vi "manual_random.vi"(8 "error in (no error)":errorcluster, 11 "data":variant) -> (0 "error out":errorcluster)   [LabVIEW 2015, in "example_01.lvlib"]
doc: "manual_random.vi will generate a random value and provide it via variant."
uses:
  example_01.lvlib
  _controls/steps_actions_data.ctl
  _controls/steps_actions.ctl
  <userlib>/antonio-alexander/lv-recipe-machine/lv-recipe-machine.lvlib
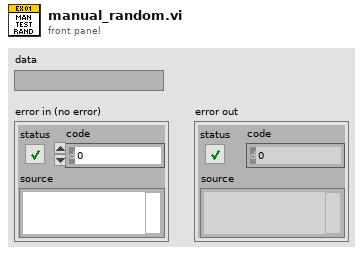
[diagram p1: front panel]
types:
  T1 = typedef "example_01.lvlib/steps_actions.ctl" = enum16{"<steps_actions>", "manual_random", "manual_comparison", "manual_wait", "auto_random", "auto_wait", "criteria_initialize", "criteria_count", "criteria_comparison", "transition_simple", "transition_count", "transition_comparison", "launch_wait", "<null>"}
  T2 = typedef "example_01.lvlib/steps_actions_data.ctl" = cluster{"step_action":T1, "data":variant}
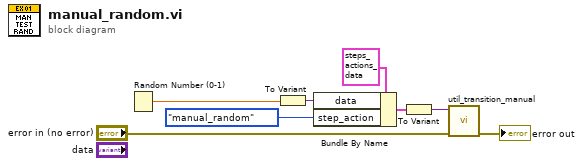
[diagram p0: block diagram]
diagram:
  n1 = Random Number (0-1)() -> (number: 0 to 1=w5:dbl)
  n2 = To Variant(anything=w5) -> (Variant=w4:variant)
  n3 = Bundle By Name(cluster=T2 {"step_action"=enum."<steps_actions>", "data"=variant}, "data"=w4, "step_action"=steps_actions."manual_random" ("manual_action")) -> (w6:T2)
  n4 = To Variant(anything=w6) -> (Variant=w3:variant)
  n5 = call <userlib>:"util_transition_manual.vi"("error in (no error)"="error in (no error)", "data"=w3) -> ("error out"=→"error out":errorcluster)  [unwired: 9 in]
